vi "RT Run FPGA VI.vi"() -> ()   [LabVIEW 2026]
uses:
  <vilib>/FPGAPlugInAG/cRIO-9047/niLvFpga_Open_cRIO-9047.vi
  <vilib>/FPGAPlugInAG/cRIO-9047/niLvFpga_Run_cRIO-9047.vi
  <vilib>/Utility/error.llb/Error Cluster From Error Code.vi
  <vilib>/rvi/errors/niLvFpgaAdjustHostInterfaceError.vi
  <vilib>/FPGAPlugInAG/cRIO-9047/niLvFpga_Reset_cRIO-9047.vi
  <vilib>/FPGAPlugInAG/cRIO-9047/niLvFpga_Close_cRIO-9047.vi
  <vilib>/rvi/interface/nirviOpenFPGA/nirviOpenFPGA.xnode
  FPGA Bitfiles/normbuttonpress_FPGATarget_FPGAVI_UBJ8qD7nAyY.lvbitx
  FPGA VI.vi
  <vilib>/rvi/interface/nirviMethod/nirviMethod.xnode
  <vilib>/rvi/interface/nirviReadWriteControl/nirviReadWriteControl.xnode
  <vilib>/rvi/interface/nirviCloseFPGA/nirviCloseFPGA.xnode
  NiFpgaLv.dll
panel:
  in  "beep duration":i32=70
  in  "# of LED's lit at once":i16=11
  in  "activation threshold":u32=250
  in  "stop":bool
  in  "PWM Speaker Freq":u16[](array[numeric])=[432, 543, 754, 865, 1087]
  out "Score":u16
  out "Time Left":dbl
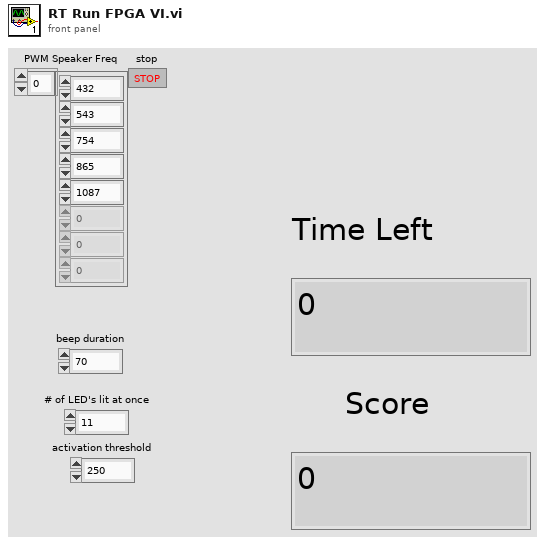
[diagram p1: front panel]
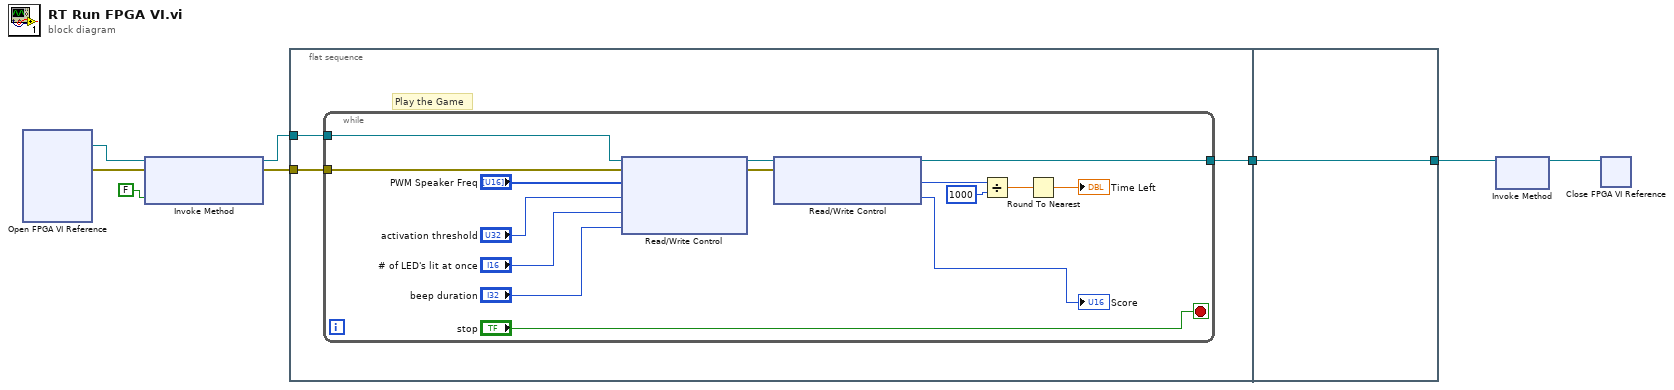
[diagram p0: block diagram]
diagram:
  n1 = xnode "Open FPGA VI Reference"() -> ("FPGA VI Reference Out"=w7:refnum<k20>, "error out"=w8:errorcluster)  [unwired: 2 in]
  n2 = xnode "Invoke Method"("FPGA VI Reference In"=w7, "error in"=w8, "Wait Until Done (F)"=FALSE) -> ("FPGA VI Reference Out"=w5:refnum<k20>, "error out"=w4:errorcluster)
  n3 = flat-sequence {
    tunnel: w5 -> [w10]
    tunnel: w4 -> [w9]
    tunnel: [w11] -> w6
    tunnel: [w27] -> w1
    tunnel: w6 -> [w27]
    frame #0 {
      # "Play the Game"
      n4 = while {
        tunnel: [w24] -> w11
        tunnel: w10 -> [w20]
        tunnel: w9 -> [w19]
        stop <- "stop" stop-if-true
        n5 = xnode "Read/Write Control"("FPGA VI Reference In"=w20, "error in"=w19, "PWM Speaker Freq"="PWM Speaker Freq", "activation threshold"="activation threshold", "# of LED's lit at once"="# of LED's lit at once", "beep duration"="beep duration") -> ("FPGA VI Reference Out"=w18:refnum<k20>, "error out"=w17:errorcluster)
        n6 = xnode "Read/Write Control"("FPGA VI Reference In"=w18, "error in"=w17) -> ("FPGA VI Reference Out"=w24:refnum<k20>, "Time Left (ms)"=w23:i32, "Score"=→"Score":u16)  [unwired: 1 out]
        n7 = Divide(x=w23, y=u32 1000 ("x")) -> (x/y=w25:dbl)
        n8 = Round To Nearest(number=w25) -> (nearest integer value=→"Time Left":dbl)
      }
    }
    frame #1 {
    }
  }
  n9 = xnode "Invoke Method"("FPGA VI Reference In"=w1) -> ("FPGA VI Reference Out"=w2:refnum<k20>)  [unwired: 1 in, 1 out]
  n10 = xnode "Close FPGA VI Reference"("FPGA VI Reference In"=w2) -> ()  [unwired: 1 in, 1 out]
